vi "global-1.vi"() -> ()   [LabVIEW 2015]
panel:
  out "496":T1
  out "管理机遥测":dbl[](array[numeric]) format="%.1f"
  out "SCADA屏通信状态":bool
  out "管理机通信状态":bool
  in  "模拟屏VISA":refnum<visa-resource-name>="COM8"
  in  "管理机VISA":refnum<visa-resource-name>="COM8"
  out "495":T2
  in  "476":T3
  in  "473":T4
  in  "472":T5
  in  "471":T6
  in  "长度1-1":T7
  in  "长度1-2":T8
  in  "长度2":T9
  # "SCADA屏幕点位"
  # "管理机"
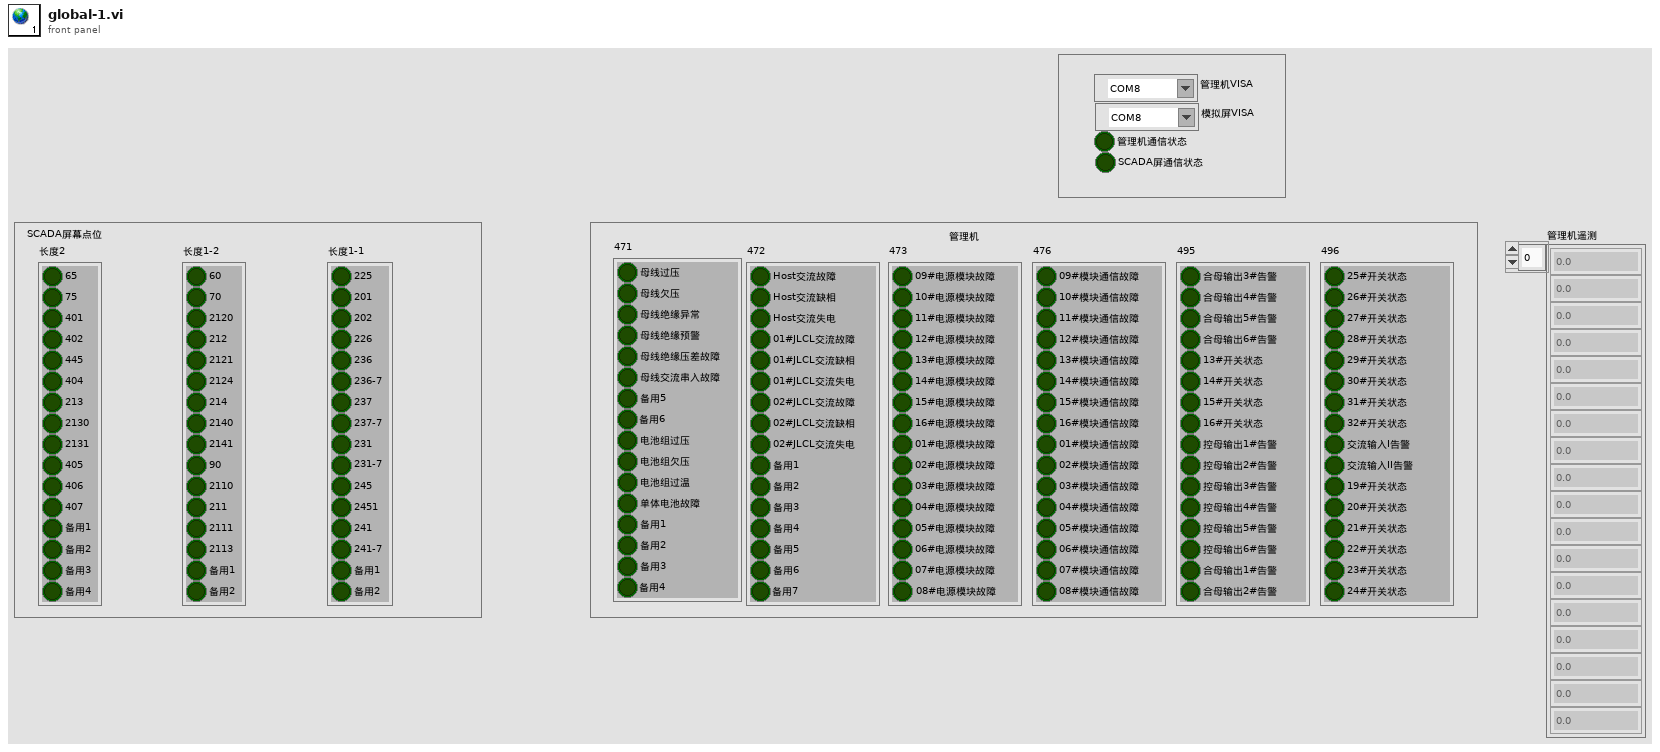
[diagram p1: front panel]
types:
  T1 = cluster{"25#开关状态":bool, "26#开关状态":bool, "27#开关状态":bool, "28#开关状态":bool, "29#开关状态":bool, "30#开关状态":bool, "31#开关状态":bool, "32#开关状态":bool, "交流输入I告警":bool, "交流输入II告警":bool, "19#开关状态":bool, "20#开关状态":bool, "21#开关状态":bool, "22#开关状态":bool, "23#开关状态":bool, "24#开关状态":bool}
  T2 = cluster{"合母输出3#告警":bool, "合母输出4#告警":bool, "合母输出5#告警":bool, "合母输出6#告警":bool, "13#开关状态":bool, "14#开关状态":bool, "15#开关状态":bool, "16#开关状态":bool, "控母输出1#告警":bool, "控母输出2#告警":bool, "控母输出3#告警":bool, "控母输出4#告警":bool, "控母输出5#告警":bool, "控母输出6#告警":bool, "合母输出1#告警":bool, "合母输出2#告警":bool}
  T3 = cluster{"09#模块通信故障":bool, "10#模块通信故障":bool, "11#模块通信故障":bool, "12#模块通信故障":bool, "13#模块通信故障":bool, "14#模块通信故障":bool, "15#模块通信故障":bool, "16#模块通信故障":bool, "01#模块通信故障":bool, "02#模块通信故障":bool, "03#模块通信故障":bool, "04#模块通信故障":bool, "05#模块通信故障":bool, "06#模块通信故障":bool, "07#模块通信故障":bool, "08#模块通信故障":bool}
  T4 = cluster{"09#电源模块故障":bool, "10#电源模块故障":bool, "11#电源模块故障":bool, "12#电源模块故障":bool, "13#电源模块故障":bool, "14#电源模块故障":bool, "15#电源模块故障":bool, "16#电源模块故障":bool, "01#电源模块故障":bool, "02#电源模块故障":bool, "03#电源模块故障":bool, "04#电源模块故障":bool, "05#电源模块故障":bool, "06#电源模块故障":bool, "07#电源模块故障":bool, " 08#电源模块故障":bool}
  T5 = cluster{"Host交流故障":bool, "Host交流缺相":bool, "Host交流失电":bool, "01#JLCL交流故障":bool, "01#JLCL交流缺相":bool, "01#JLCL交流失电":bool, "02#JLCL交流故障":bool, "02#JLCL交流缺相":bool, "02#JLCL交流失电":bool, "备用1":bool, "备用2":bool, "备用3":bool, "备用4":bool, "备用5":bool, "备用6":bool, " 备用7":bool}
  T6 = cluster{"母线过压":bool, "母线欠压":bool, "母线绝缘异常":bool, "母线绝缘预警":bool, "母线绝缘压差故障":bool, "母线交流串入故障":bool, "备用5":bool, " 备用6":bool, "电池组过压":bool, "电池组欠压":bool, "电池组过温":bool, "单体电池故障":bool, "备用1":bool, "备用2":bool, "备用3":bool, " 备用4":bool}
  T7 = cluster{"225":bool, "201":bool, "202":bool, "226":bool, "236":bool, "236-7":bool, "237":bool, "237-7":bool, "231":bool, "231-7":bool, "245":bool, "2451":bool, "241":bool, "241-7":bool, "备用1":bool, "备用2":bool}
  T8 = cluster{"60":bool, "70":bool, "2120":bool, "212":bool, "2121":bool, "2124":bool, "214":bool, "2140":bool, "2141":bool, "90":bool, "2110":bool, "211":bool, "2111":bool, "2113":bool, "备用1":bool, "备用2":bool}
  T9 = cluster{"65":bool, "75":bool, "401":bool, "402":bool, "445":bool, "404":bool, "213":bool, "2130":bool, "2131":bool, "405":bool, "406":bool, "407":bool, "备用1":bool, "备用2":bool, "备用3":bool, "备用4":bool}
diagram:
